vi "ManipEnd.vi"() -> (0 "Error Out":errorcluster, 1 "Advance Trigger":bool)   [LabVIEW 2020]
doc: "Stops the manipulator sequencer.\n\nParameters: None"
uses:
  GlobalAutonomous.vi
  GlobalDriverStationCommands.vi
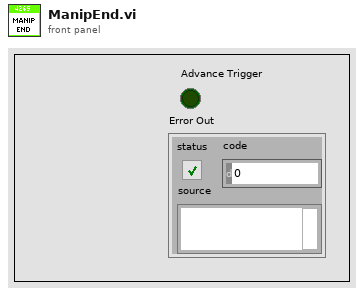
[diagram p1: front panel]
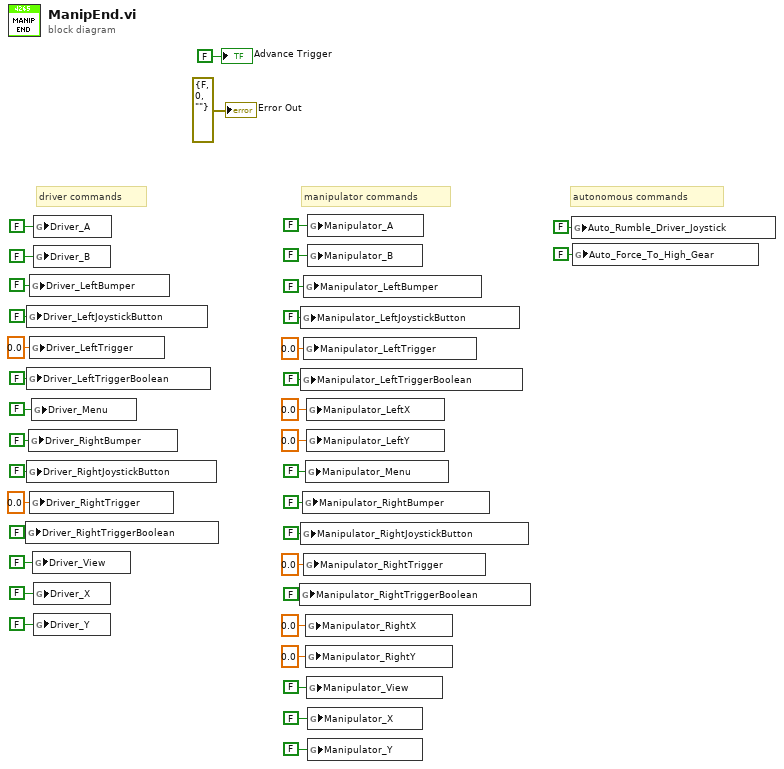
[diagram p0: block diagram]
diagram:
  # "manipulator commands"
  # "driver commands"
  # "autonomous commands"
  n1 = global write "GlobalDriverStationCommands.vi" "Driver_RightTriggerBoolean"(FALSE ("Driver_RightTriggerBoolean")) -> ()
  n2 = global write "GlobalDriverStationCommands.vi" "Driver_LeftJoystickButton"(FALSE ("Driver_LeftJoystickButton")) -> ()
  n3 = global write "GlobalDriverStationCommands.vi" "Driver_LeftTriggerBoolean"(FALSE ("Driver_LeftTriggerBoolean")) -> ()
  n4 = global write "GlobalDriverStationCommands.vi" "Driver_RightJoystickButton"(FALSE ("Driver_RightJoystickButton")) -> ()
  n5 = global write "GlobalDriverStationCommands.vi" "Driver_RightBumper"(FALSE ("Driver_RightBumper")) -> ()
  n6 = global write "GlobalDriverStationCommands.vi" "Driver_LeftBumper"(FALSE ("Driver_LeftBumper")) -> ()
  n7 = global write "GlobalDriverStationCommands.vi" "Driver_LeftTrigger"(0.0 ("Driver_LeftTrigger")) -> ()
  n8 = global write "GlobalDriverStationCommands.vi" "Driver_RightTrigger"(0.0 ("Driver_RightTrigger")) -> ()
  n9 = global write "GlobalDriverStationCommands.vi" "Driver_Menu"(FALSE ("Driver_Menu")) -> ()
  n10 = global write "GlobalDriverStationCommands.vi" "Driver_View"(FALSE ("Driver_View")) -> ()
  n11 = global write "GlobalDriverStationCommands.vi" "Driver_A"(FALSE ("Driver_A")) -> ()
  n12 = global write "GlobalDriverStationCommands.vi" "Driver_B"(FALSE ("Driver_B")) -> ()
  n13 = global write "GlobalDriverStationCommands.vi" "Driver_X"(FALSE ("Driver_X")) -> ()
  n14 = global write "GlobalDriverStationCommands.vi" "Driver_Y"(FALSE ("Driver_Y")) -> ()
  n15 = global write "GlobalDriverStationCommands.vi" "Manipulator_RightTriggerBoolean"(FALSE ("Driver_RightTriggerBoolean")) -> ()
  n16 = global write "GlobalDriverStationCommands.vi" "Manipulator_LeftJoystickButton"(FALSE ("Driver_LeftJoystickButton")) -> ()
  n17 = global write "GlobalDriverStationCommands.vi" "Manipulator_LeftTriggerBoolean"(FALSE ("Driver_LeftTriggerBoolean")) -> ()
  n18 = global write "GlobalDriverStationCommands.vi" "Manipulator_RightJoystickButton"(FALSE ("Driver_RightJoystickButton")) -> ()
  n19 = global write "GlobalDriverStationCommands.vi" "Manipulator_RightBumper"(FALSE ("Driver_RightBumper")) -> ()
  n20 = global write "GlobalDriverStationCommands.vi" "Manipulator_LeftBumper"(FALSE ("Driver_LeftBumper")) -> ()
  n21 = global write "GlobalDriverStationCommands.vi" "Manipulator_LeftTrigger"(0.0 ("Driver_LeftTrigger")) -> ()
  n22 = global write "GlobalDriverStationCommands.vi" "Manipulator_RightTrigger"(0.0 ("Driver_RightTrigger")) -> ()
  n23 = global write "GlobalDriverStationCommands.vi" "Manipulator_Menu"(FALSE ("Driver_Menu")) -> ()
  n24 = global write "GlobalDriverStationCommands.vi" "Manipulator_RightX"(0.0 ("Driver_RightX")) -> ()
  n25 = global write "GlobalDriverStationCommands.vi" "Manipulator_RightY"(0.0 ("Driver_RightY")) -> ()
  n26 = global write "GlobalDriverStationCommands.vi" "Manipulator_LeftX"(0.0 ("Driver_LeftX")) -> ()
  n27 = global write "GlobalDriverStationCommands.vi" "Manipulator_LeftY"(0.0 ("Driver_LeftY")) -> ()
  n28 = global write "GlobalDriverStationCommands.vi" "Manipulator_View"(FALSE ("Driver_View")) -> ()
  n29 = global write "GlobalDriverStationCommands.vi" "Manipulator_A"(FALSE ("Driver_A")) -> ()
  n30 = global write "GlobalDriverStationCommands.vi" "Manipulator_B"(FALSE ("Driver_B")) -> ()
  n31 = global write "GlobalDriverStationCommands.vi" "Manipulator_X"(FALSE ("Driver_X")) -> ()
  n32 = global write "GlobalDriverStationCommands.vi" "Manipulator_Y"(FALSE ("Driver_Y")) -> ()
  n33 = global write "GlobalAutonomous.vi" "Auto_Rumble_Driver_Joystick"(FALSE ("Auto_Force_To_Low_Gear")) -> ()
  n34 = global write "GlobalAutonomous.vi" "Auto_Force_To_High_Gear"(FALSE ("Auto_Force_To_Low_Gear")) -> ()
  "Advance Trigger" <- FALSE ("Advance Trigger")
  "Error Out" <- errorcluster {"status"=FALSE, "code"=0, "source"=""} ("error constant")
